vi "PositionerCapture_FocusedGaussLaw.vi"() -> ()   [LabVIEW 2011]
doc: "CONEX - CC Virtual Front Panel:\n\nThis is a sample of an application that can be built with the LabVIEW drivers.\n\nPress HOME / ENABLE in top left of panel to put stage in Ready state for motion."
uses:
  <vilib>/userDefined/High Color/IMAQdx.ctl
  <vilib>/Platform/TimedLoop/XDataNode/timing_clust.ctl
  <vilib>/Platform/TimedLoop/XDataNode/nitl_modes.ctl
  <vilib>/Platform/TimedLoop/XDataNode/wakeup.ctl
  <vilib>/Platform/TimedLoop/XDataNode/XDataNode.xnode
  <vilib>/Platform/TimedLoop/XDataNode/XDNodeRunTimeDep.lvlib
  <vilib>/vision/driver/NI_Vision_Acquisition_Software.lvlib
panel:
  out "Phase":bool
  out "Amp":bool
  in  "Next":bool
  out "Current noUnits":dbl caption="mm" format="%#_6f"
  in  "lambda":dbl caption="nm" format="%#_6f"
  in  "Units":string(combo)="mm"
  in  "Go0":bool
  in  "Zero position":dbl caption="mm" format="%#_6f"
  in  "Tare":bool
  out "Relative position":dbl caption="mm" format="%#_6f"
  in  "Folder's path where save the captures":path
  out "Image":T1(plugin-control)
  in  "(1) Go to:":dbl=1.0 caption="mm"
  out "Title":string
  in  "Set Max":bool
  in  "Set Min":bool
  in  "Max":dbl
  in  "Min":dbl
  in  "Set velocity":bool
  out "Stop cycle":bool=TRUE
  out "Title 2":string
  in  "Cycle":bool
  in  "Go2":bool
  in  "Go1":bool
  in  "(2) Go to:":dbl=1.0 caption="mm"
  in  "-":bool
  in  "+":bool
  in  "Step:":dbl caption="mm" format="%#_6f"
  out "Position History":dbl(graph)=1.5
  in  "Action":bool
  out "Stop polling":bool=TRUE
  out "Controller state description":string="STATUS"
  out "Velocity MAX":dbl=0.4
  out "Controller state":string="33"
  out "Positioner error":string="0000"
  in  "Velocity:":dbl format="%#_6f"
  in  "Exit":bool=TRUE
  out "Target position":dbl
  in  "Exit":bool
  in  "Position glissière":cluster{dbl, dbl}(slide) scale=0.0..25.0
  out "Current position":dbl caption="mm" format="%#_6f"
  # "mm/s"
  # "mm"
  # "Limits:"
  # "mm"
  # "(1)"
  # "(2)"
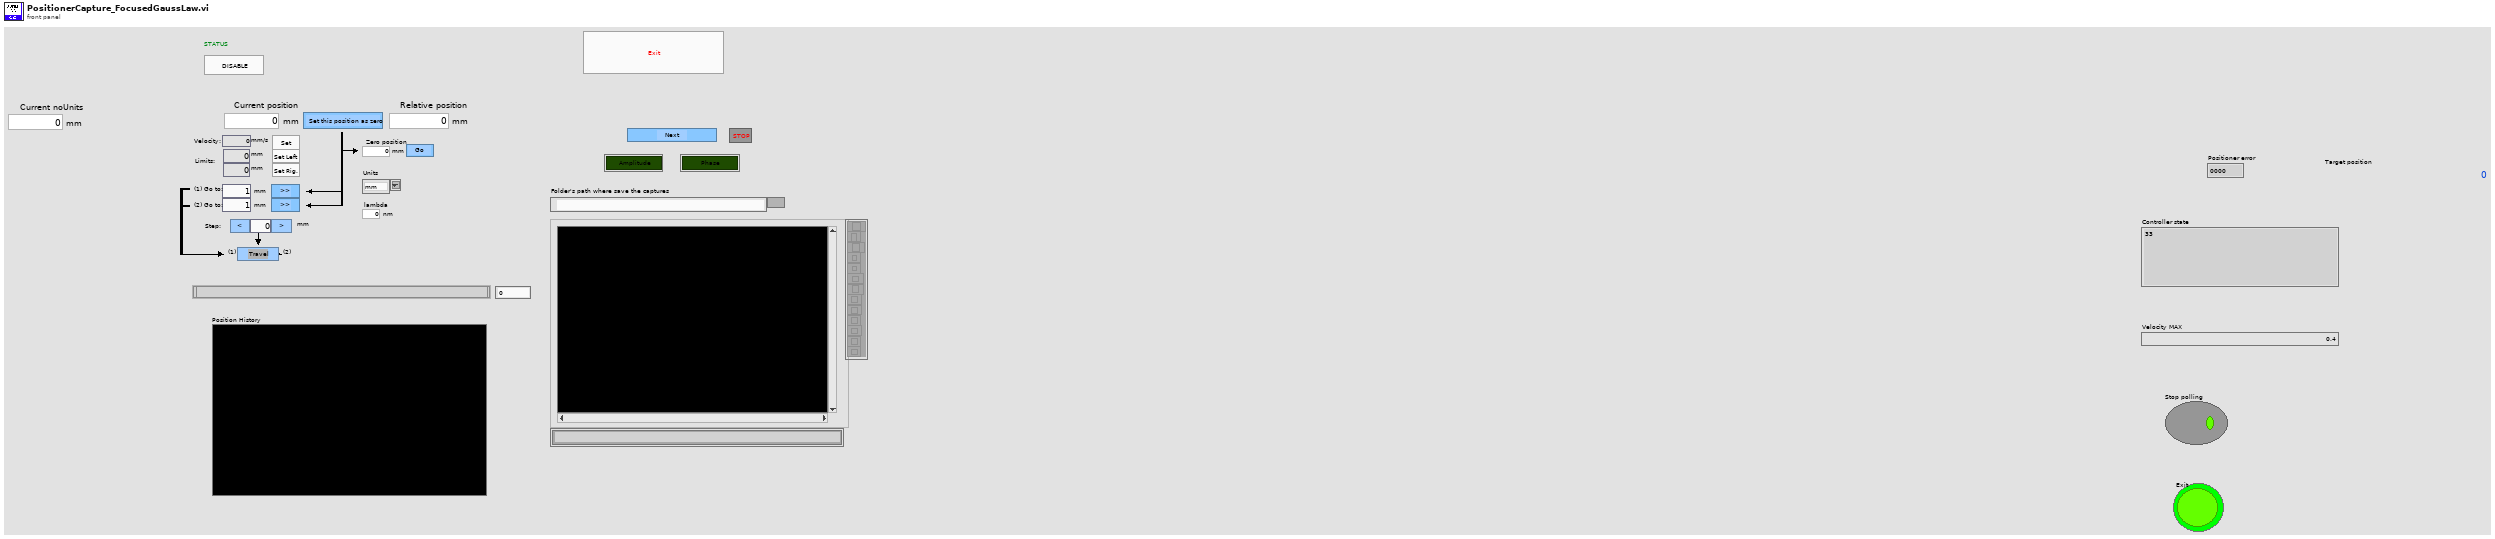
[diagram p1: front panel]
types:
  T1 = typedef "IMAQ Image.ctl" = refnum<image>
  T2 = typedef "IMAQdx.ctl" = refnum<k21>
  T3 = typedef "XDNodeRunTimeDep.lvlib/timing_clust.ctl" = cluster{"Expected End [f-1]":u64, "Actual End [f-1]":u64, "Finished Late? [f-1]":bool, "Expected End [i-1]":u64, "Actual End [i-1]":u64, "Finished Late? [i-1]":bool, "Expected Start [i]":u64, "Actual Start [i]":u64, "Expected Start [f]":u64, "Actual Start [f]":u64, "Source Name":string, "Structure Name":string, "Period":i64, "Deadline":i64, "Offset":i64, "Start":i64, "Priority":i32, "Timeout":i32, "Mode":T4, "Wakeup Reason":T5, "Error":errorcluster, "Source Type":string, "Secondary Source Type":string, "Global End Time":u64, "Global Start Time":u64, "Frame Duration":u64, "Iteration Duration":u64, "Assigned CPU":i32, "I/O Scan Engine Mode":u32}
  T4 = typedef "XDNodeRunTimeDep.lvlib/nitl_modes.ctl" = enum32{"No Change", "Process missed periods, maintain original phase", "Discard missed periods, maintain original phase", "Process missed periods, ignore original phase", "Discard missed periods, ignore original phase"}
  T5 = typedef "XDNodeRunTimeDep.lvlib/wakeup.ctl" = enum32{"Normal", "Aborted", "Asynchronous wakeup", "Timing source error", "Timed loop error", "Timeout"}
  T6 = cluster{"VISA resource name":refnum<visa-resource-name>, "Device name":string, "Controller address":i32, "error":errorcluster}
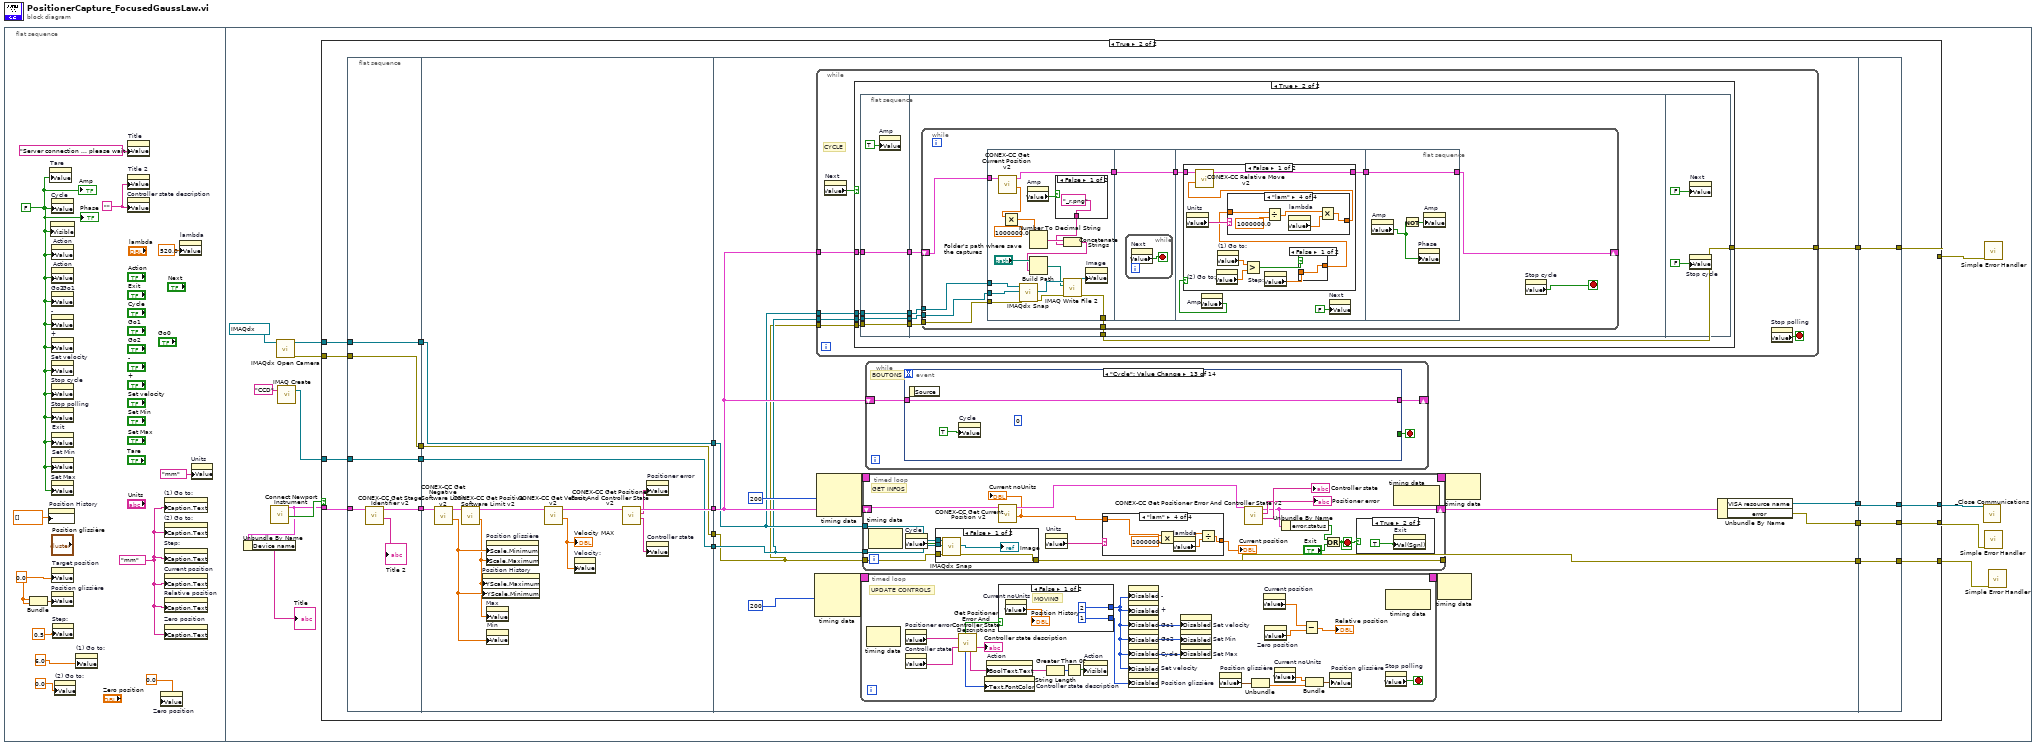
[diagram p0: block diagram]
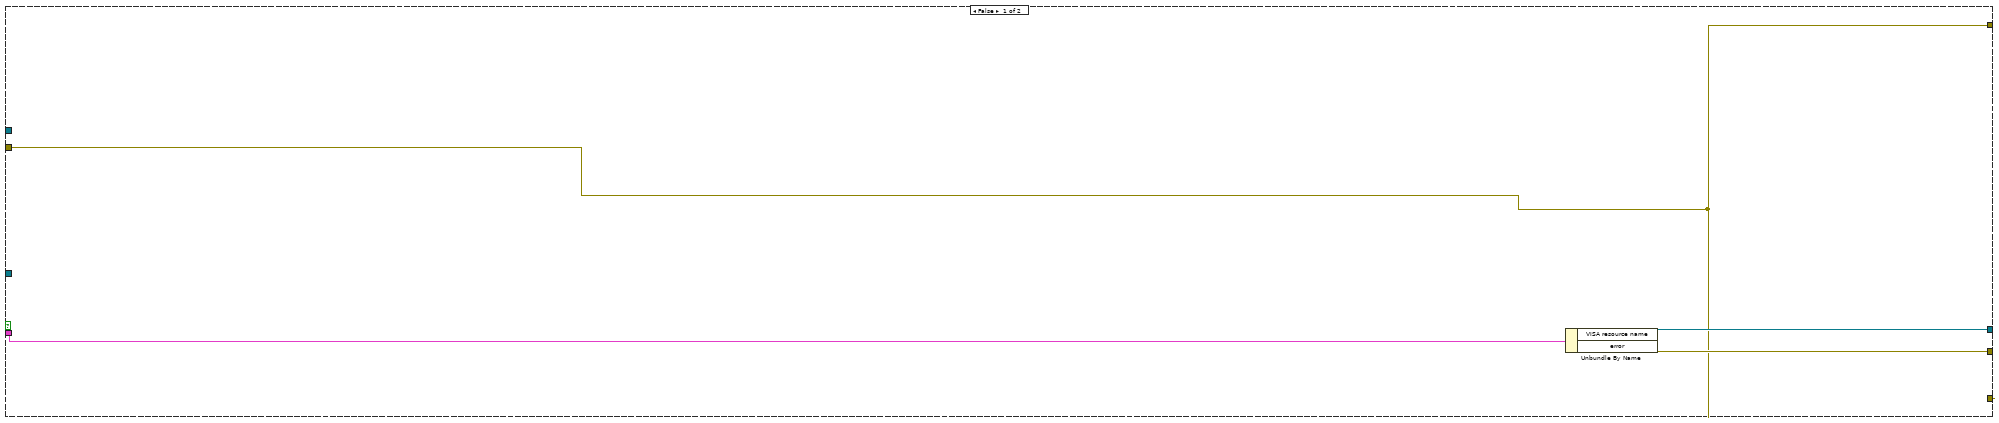
[diagram p2: hidden frame]
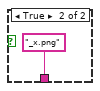
[diagram p4: hidden frame]
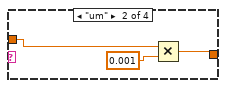
[diagram p6: hidden frame]
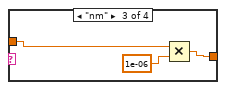
[diagram p7: hidden frame]
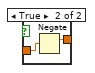
[diagram p8: hidden frame]
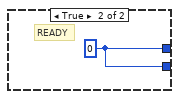
[diagram p10: hidden frame]
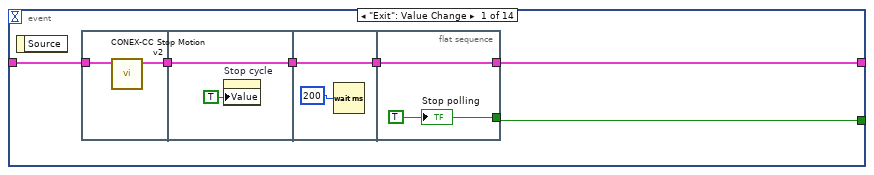
[diagram p11: hidden frame]
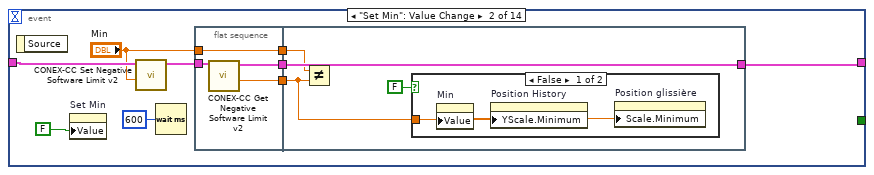
[diagram p12: hidden frame]
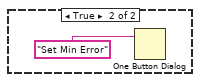
[diagram p13: hidden frame]
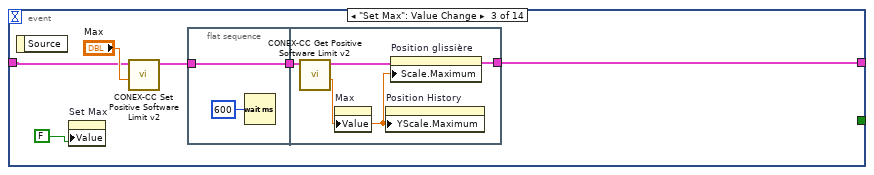
[diagram p14: hidden frame]
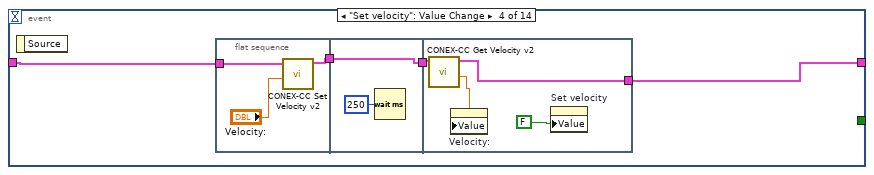
[diagram p15: hidden frame]
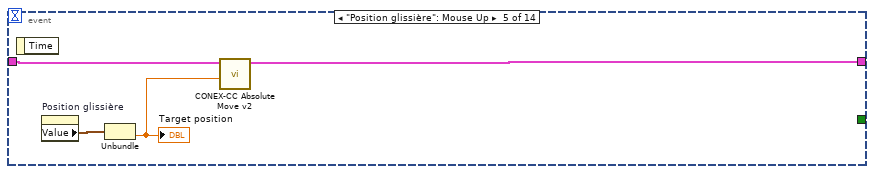
[diagram p16: hidden frame]
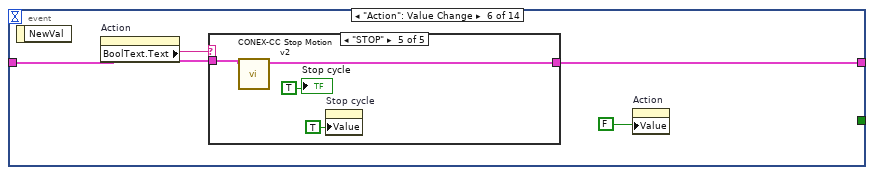
[diagram p17: hidden frame]
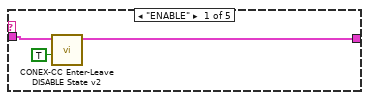
[diagram p18: hidden frame]
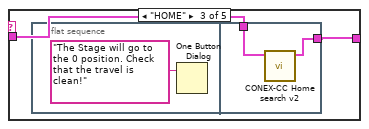
[diagram p20: hidden frame]
diagram:
  n1 = flat-sequence {
    frame #0 {
      w3 = "mm" ("Units")
      w1 = FALSE
      w12 = 0.0
      w11 = ""
      n2 = Bundle(w12, w12) -> (w13:cluster{dbl, dbl})  [unwired: 1 out]
      n3 = property on="Position History" class="WFChart (strict)"("History Data"=dbl[] [] ("Données d'historique")) -> ()  [unwired: 2 in, 2 out]
      n4 = property on="Tare" class="Bool (strict)"("Value"=w1) -> ()  [unwired: 2 in, 2 out]
      n5 = property on="Action" class="Bool (strict)"("Visible"=w1) -> ()  [unwired: 2 in, 2 out]
      n6 = property on="Cycle" class="Bool (strict)"("Value"=w1) -> ()  [unwired: 2 in, 2 out]
      n7 = property on="Action" class="Bool (strict)"("Value"=w1) -> ()  [unwired: 2 in, 2 out]
      n8 = property on="Go1" class="Bool (strict)"("Value"=w1) -> ()  [unwired: 2 in, 2 out]
      n9 = property on="Go2" class="Bool (strict)"("Value"=w1) -> ()  [unwired: 2 in, 2 out]
      n10 = property on="-" class="Bool (strict)"("Value"=w1) -> ()  [unwired: 2 in, 2 out]
      n11 = property on="+" class="Bool (strict)"("Value"=w1) -> ()  [unwired: 2 in, 2 out]
      n12 = property on="Set velocity" class="Bool (strict)"("Value"=w1) -> ()  [unwired: 2 in, 2 out]
      n13 = property on="Stop cycle" class="Bool (strict)"("Value"=w1) -> ()  [unwired: 2 in, 2 out]
      n14 = property on="Stop polling" class="Bool (strict)"("Value"=w1) -> ()  [unwired: 2 in, 2 out]
      n15 = property on="Exit" class="Bool (strict)"("Value"=w1) -> ()  [unwired: 2 in, 2 out]
      n16 = property on="Set Min" class="Bool (strict)"("Value"=w1) -> ()  [unwired: 2 in, 2 out]
      n17 = property on="Set Max" class="Bool (strict)"("Value"=w1) -> ()  [unwired: 2 in, 2 out]
      n18 = property on="Target position" class="DigNum (strict)"("Value"=w12) -> ()  [unwired: 2 in, 2 out]
      n19 = property on="Position glissière" class="Slide (strict)"("Value"=w13) -> ()  [unwired: 2 in, 2 out]
      n20 = property on="Step:" class="DigNum (strict)"("Value"=0.5 ("Step")) -> ()  [unwired: 2 in, 2 out]
      n21 = property on="(2) Go to:" class="DigNum (strict)"("Value"=0.0 ("Abs. Move 2")) -> ()  [unwired: 2 in, 2 out]
      n22 = property on="(1) Go to:" class="DigNum (strict)"("Value"=6.0 ("Abs. Move 1")) -> ()  [unwired: 2 in, 2 out]
      n23 = property on="Title" class="Str"("Value"="Server connection ... please wait." ("Title")) -> ()  [unwired: 2 in, 2 out]
      n24 = property on="Title 2" class="Str"("Value"=w11) -> ()  [unwired: 2 in, 2 out]
      n25 = property on="Controller state description" class="Str"("Value"=w11) -> ()  [unwired: 2 in, 2 out]
      n26 = property on="Zero position" class="DigNum (strict)"("Value"=0.0 ("Zero position")) -> ()  [unwired: 2 in, 2 out]
      n27 = property on="(1) Go to:" class="DigNum (strict)"("Caption.Text"=w3) -> ()  [unwired: 2 in, 2 out]
      n28 = property on="(2) Go to:" class="DigNum (strict)"("Caption.Text"=w3) -> ()  [unwired: 2 in, 2 out]
      n29 = property on="Step:" class="DigNum (strict)"("Caption.Text"=w3) -> ()  [unwired: 2 in, 2 out]
      n30 = property on="Current position" class="DigNum (strict)"("Caption.Text"=w3) -> ()  [unwired: 2 in, 2 out]
      n31 = property on="Relative position" class="DigNum (strict)"("Caption.Text"=w3) -> ()  [unwired: 2 in, 2 out]
      n32 = property on="Zero position" class="DigNum (strict)"("Caption.Text"=w3) -> ()  [unwired: 2 in, 2 out]
      n33 = property on="lambda" class="DigNum (strict)"("Value"=520.0 ("lambda")) -> ()  [unwired: 2 in, 2 out]
      n34 = property on="Units" class="CmbBox"("Value"="mm" ("Units")) -> ()  [unwired: 2 in, 2 out]
      "Amp" <- w1
      "Phase" <- w1
    }
    frame #1 {
      n35 = call <userlib>:"Connect Newport Instrument.vi"() -> ("Connected"=w23:bool, "Device Connection Cluster"=w22:T6)  [unwired: 7 in, 3 out]
      n36 = Unbundle By Name(w22) -> ("Device name"=→"Title":string)
      n37 = call <vilib>:"IMAQdx Open Camera.vi"("Session In"=T2 "Paraxial") -> ("error out"=w16:errorcluster, "Session Out"=w18:T2)  [unwired: 9 in]
      n38 = call "IMAQ Create"("Image Name"="CCD") -> ("New Image"=w17:T1)  [unwired: 4 in, 1 out]
      n39 = case shown="True" w23 {
        tunnel: [w28 w49] -> w25
        tunnel: w22 -> [w29 w47]
        tunnel: [w27 w43] -> w21
        tunnel: w18 -> [_ w41]
        tunnel: w17 -> [_ w38]
        tunnel: w16 -> [w26 w35]
        tunnel: [w26 w32] -> w15
        tunnel: [w26 w30] -> w14
        frame False {
          n40 = Unbundle By Name(w29) -> ("VISA resource name"=w27:refnum<visa-resource-name>, "error"=w28:errorcluster)
        }
        frame True {
          n41 = flat-sequence {
            tunnel: w47 -> [w55]
            tunnel: [w53] -> w46
            tunnel: [w52] -> w42
            tunnel: w41 -> [w52]
            tunnel: [w51] -> w39
            tunnel: w38 -> [w51]
            tunnel: [w50] -> w36
            tunnel: w35 -> [w50]
            tunnel: [w65] -> w48
            tunnel: w46 -> [w62]
            tunnel: w42 -> [w58]
            tunnel: [w58] -> w40
            tunnel: w39 -> [w57]
            tunnel: [w57] -> w37
            tunnel: w36 -> [w56]
            tunnel: [w56] -> w34
            tunnel: w48 -> [w74]
            tunnel: [w76] -> w45
            tunnel: [w75] -> w44
            tunnel: w40 -> [w73]
            tunnel: w37 -> [w72]
            tunnel: w34 -> [w71]
            tunnel: [w70] -> w33
            tunnel: [w69] -> w31
            tunnel: [w449] -> w49
            tunnel: w45 -> [w448]
            tunnel: w44 -> [w449]
            tunnel: [w448] -> w43
            tunnel: [w447] -> w32
            tunnel: w33 -> [w447]
            tunnel: [w446] -> w30
            tunnel: w31 -> [w446]
            frame #0 {
              n42 = call <userlib>:"CONEX-CC Get Stage Identifier v2.vi"("Connection Cluster in"=w55) -> ("Identifier"=→"Title 2":string, "Connection Cluster out"=w53:T6)  [unwired: 9 in]
            }
            frame #1 {
              n43 = call <userlib>:"CONEX-CC Get Negative Software Limit v2.vi"("Connection Cluster in"=w62) -> ("Left limit"=w67:dbl, "Connection Cluster out"=w61:T6)  [unwired: 9 in]
              n44 = call <userlib>:"CONEX-CC Get Positive Software Limit v2.vi"("Connection Cluster in"=w61) -> ("Right limit"=w66:dbl, "Connection Cluster out"=w60:T6)  [unwired: 9 in]
              n45 = property on="Position History" class="WFChart (strict)"("YScale.Maximum"=w66, "YScale.Minimum"=w67) -> ()  [unwired: 2 in, 2 out]
              n46 = property on="Position glissière" class="Slide (strict)"("Scale.Minimum"=w67, "Scale.Maximum"=w66) -> ()  [unwired: 2 in, 2 out]
              n47 = property on="Max" class="DigNum (strict)"("Value"=w66) -> ()  [unwired: 2 in, 2 out]
              n48 = property on="Min" class="DigNum (strict)"("Value"=w67) -> ()  [unwired: 2 in, 2 out]
              n49 = call <userlib>:"CONEX-CC Get Velocity v2.vi"("Connection Cluster in"=w60) -> ("Velocity"=w68:dbl, "Connection Cluster out"=w59:T6)  [unwired: 8 in, 1 out]
              "Velocity MAX" <- w68
              n50 = property on="Velocity:" class="DigNum (strict)"("Value"=w68) -> ()  [unwired: 2 in, 2 out]
              n51 = call <userlib>:"CONEX-CC Get Positioner Error And Controller State v2.vi"("Connection Cluster in"=w59) -> ("Controller state"=w63:string, "Positioner error"=w64:string, "Connection Cluster out"=w65:T6)  [unwired: 8 in]
              n52 = property on="Positioner error" class="Str"("Value"=w64) -> ()  [unwired: 2 in, 2 out]
              n53 = property on="Controller state" class="Str"("Value"=w63) -> ()  [unwired: 2 in, 2 out]
            }
            frame #2 {
              n54 = node-c288(i64 200 ("Période")) -> (w81:T3)  [unwired: 1 in, 1 out]
              n55 = while {
                tunnel: w74 -> [w90]
                tunnel: w73 -> [w87]
                tunnel: w72 -> [w86]
                tunnel: w71 -> [w85]
                tunnel: [w84] -> w69
                stop <- w89 stop-if-true
                # "CYCLE"
                n56 = property on="Next" class="Bool (strict)"() -> ("Value"=w88:bool)  [unwired: 2 in, 2 out]
                n57 = case shown="True" w88 {
                  tunnel: w90 -> [_ w97]
                  tunnel: w87 -> [_ w100]
                  tunnel: w86 -> [_ w99]
                  tunnel: w85 -> [w91 w98]
                  tunnel: [w91 w96] -> w84
                  frame False {
                  }
                  frame True {
                    n58 = flat-sequence {
                      tunnel: w97 -> [w102]
                      tunnel: w98 -> [w103]
                      tunnel: w99 -> [w104]
                      tunnel: w100 -> [w105]
                      tunnel: [w105] -> w95
                      tunnel: [w104] -> w94
                      tunnel: [w103] -> w93
                      tunnel: [w102] -> w92
                      tunnel: [w106] -> w96
                      tunnel: w95 -> [w110]
                      tunnel: w94 -> [w109]
                      tunnel: w93 -> [w108]
                      tunnel: w92 -> [w107]
                      frame #0 {
                        n59 = property on="Amp" class="Bool (strict)"("Value"=TRUE ("Amp")) -> ()  [unwired: 2 in, 2 out]
                      }
                      frame #1 {
                        n60 = while {
                          shift-right: [w112] -> _
                          shift-left: w107 -> [w120]
                          tunnel: w110 -> [w119]
                          tunnel: w109 -> [w115]
                          tunnel: w108 -> [w118]
                          tunnel: [w113] -> w106
                          stop <- w111 stop-if-true
                          n61 = flat-sequence {
                            tunnel: w120 -> [w132]
                            tunnel: w119 -> [w130]
                            tunnel: w115 -> [w129]
                            tunnel: w118 -> [w128]
                            tunnel: [w131] -> w116
                            tunnel: [w121] -> w113
                            tunnel: [w141] -> w117
                            tunnel: w116 -> [w141]
                            tunnel: w117 -> [w146]
                            tunnel: [w145] -> w114
                            tunnel: [w174] -> w112
                            tunnel: w114 -> [w174]
                            frame #0 {
                              n62 = call <userlib>:"CONEX-CC Get Current Position v2.vi"("Connection Cluster in"=w132) -> ("Current position"=w124:dbl, "Connection Cluster out"=w131:T6)  [unwired: 8 in, 1 out]
                              n63 = Multiply(x=w124, y=1000000.0) -> (x*y=w137:dbl)
                              n64 = call <vilib>:"IMAQdx Snap.vi"("error in"=w128, "Image In"=w129, "Session In"=w130) -> ("error out"=w127:errorcluster, "Image Out"=w133:T1)  [unwired: 6 in, 1 out]
                              n65 = property on="Amp" class="Bool (strict)"() -> ("Value"=w123:bool)  [unwired: 2 in, 2 out]
                              n66 = Number To Decimal String(number=w137) -> (decimal integer string=w138:string)  [unwired: 1 in]
                              n67 = case shown="False" w123 {
                                tunnel: ["_r.png" ("string") "_x.png" ("string")] -> w122
                                frame False {
                                }
                                frame True {
                                }
                              }
                              n68 = Concatenate Strings(w138, w122) -> (w125:string)
                              n69 = Build Path(base path="Folder's path where save the captures", name or relative path=w125) -> (appended path=w126:path)
                              n70 = call-poly "IMAQ Write File 2"("error in (no error)"=w127, "File Path"=w126, "Image"=w133) -> ("error out"=w121:errorcluster, "Image Out (duplicate)"=w134:T1)  [unwired: 7 in]
                              n71 = property on="Image" class="ImageControl"("Value"=w134) -> ()  [unwired: 2 in, 2 out]
                            }
                            frame #1 {
                              n72 = while {
                                stop <- w142 stop-if-true
                                n73 = property on="Next" class="Bool (strict)"() -> ("Value"=w142:bool)  [unwired: 2 in, 2 out]
                              }
                            }
                            frame #2 {
                              n74 = property on="Amp" class="Bool (strict)"() -> ("Value"=w143:bool)  [unwired: 2 in, 2 out]
                              n75 = case shown="False" w143 {
                                tunnel: w146 -> [w149 w171]
                                tunnel: [w148 w171] -> w145
                                frame False {
                                n76 = property on="Units" class="CmbBox"() -> ("Value"=w155:string)  [unwired: 2 in, 2 out]
                                n77 = property on="(2) Go to:" class="DigNum (strict)"() -> ("Value"=w150:dbl)  [unwired: 2 in, 2 out]
                                n78 = property on="(1) Go to:" class="DigNum (strict)"() -> ("Value"=w151:dbl)  [unwired: 2 in, 2 out]
                                n79 = Greater?(x=w151, y=w150) -> (0:w152:bool)
                                n80 = property on="Step:" class="DigNum (strict)"() -> ("Value"=w153:dbl)  [unwired: 2 in, 2 out]
                                n81 = case shown="False" w152 {
                                tunnel: [w168 w169] -> w154
                                tunnel: w153 -> [w168 w170]
                                frame False {
                                }
                                frame True {
                                n82 = Negate(x=w170) -> (-x=w169:dbl)
                                }
                                }
                                n83 = case shown="\"lam\"" w155 {
                                tunnel: [w156 w158 w161 w164] -> w147
                                tunnel: w154 -> [w156 w157 w160 w163]
                                frame "mm", Default {
                                }
                                frame "um" {
                                n84 = Multiply(x=w157, y=0.001) -> (x*y=w158:dbl)
                                }
                                frame "nm" {
                                n85 = Multiply(x=w160, y=1e-06) -> (x*y=w161:dbl)
                                }
                                frame "lam" {
                                n86 = Divide(x=w163, y=1000000.0) -> (x/y=w166:dbl)
                                n87 = property on="lambda" class="DigNum (strict)"() -> ("Value"=w165:dbl)  [unwired: 2 in, 2 out]
                                n88 = Multiply(x=w166, y=w165) -> (x*y=w164:dbl)
                                }
                                }
                                n89 = call <userlib>:"CONEX-CC Relative Move v2.vi"("Relative displacement"=w147, "Connection Cluster in"=w149) -> ("Connection Cluster out"=w148:T6)  [unwired: 9 in]
                                }
                                frame True {
                                }
                              }
                              n90 = property on="Next" class="Bool (strict)"("Value"=FALSE ("Next")) -> ()  [unwired: 2 in, 2 out]
                            }
                            frame #3 {
                              n91 = property on="Amp" class="Bool (strict)"() -> ("Value"=w173:bool)  [unwired: 2 in, 2 out]
                              n92 = Not(x=w173) -> (.not. x?=w172:bool)
                              n93 = property on="Phase" class="Bool (strict)"("Value"=w173) -> ()  [unwired: 2 in, 2 out]
                              n94 = property on="Amp" class="Bool (strict)"("Value"=w172) -> ()  [unwired: 2 in, 2 out]
                            }
                          }
                          n95 = property on="Stop cycle" class="Bool (strict)"() -> ("Value"=w111:bool)  [unwired: 2 in, 2 out]
                        }
                      }
                      frame #2 {
                        n96 = property on="Next" class="Bool (strict)"("Value"=FALSE ("Cycle")) -> ()  [unwired: 2 in, 2 out]
                        n97 = property on="Stop cycle" class="Bool (strict)"("Value"=FALSE ("Cycle")) -> ()  [unwired: 2 in, 2 out]
                      }
                    }
                  }
                }
                n98 = property on="Stop polling" class="Bool (strict)"() -> ("Value"=w89:bool)  [unwired: 2 in, 2 out]
              }
              n99 = node-c288(i64 200 ("Période")) -> (w83:T3)  [unwired: 1 in, 1 out]
              n100 = timed-loop {
                timing: w81 -> [_]
                timing-out: [_] -> w80
                stop <- w185 stop-if-true
                # "UPDATE CONTROLS"
                n101 = node-c288() -> ()  [unwired: 2 out]
                n102 = property on="Positioner error" class="Str"() -> ("Value"=w194:string)  [unwired: 2 in, 2 out]
                n103 = property on="Controller state" class="Str"() -> ("Value"=w193:string)  [unwired: 2 in, 2 out]
                n104 = call <userlib>:"Get Positioner Error And Controller State Descriptions.vi"("Controller state"=w193, "Positioner error"=w194) -> ("Color"=w191:u32, "Action name"=w190:string, "Controller state description"=→"Controller state description":string, "IsReady?"=w187:bool)  [unwired: 2 out]
                n105 = property on="Controller state description" class="Str"("Text.FontColor"=w191) -> ()  [unwired: 2 in, 2 out]
                n106 = property on="Action" class="Bool (strict)"("BoolText.Text"=w190) -> ()  [unwired: 2 in, 2 out]
                n107 = case shown="False" w187 {
                  tunnel: [u8 2 w198] -> w184
                  tunnel: [u8 1 w198] -> w186
                  frame False {
                    # "MOVING"
                    n108 = property on="Current noUnits" class="DigNum (strict)"() -> ("Value"=→"Position History":dbl)  [unwired: 2 in, 2 out]
                  }
                  frame True {
                    w198 = u8 0
                    # "READY"
                  }
                }
                n109 = String Length(string=w190) -> (length=w189:i32)
                n110 = Greater Than 0?(x=w189) -> (x > 0?=w188:bool)
                n111 = property on="Action" class="Bool (strict)"("Visible"=w188) -> ()  [unwired: 2 in, 2 out]
                n112 = property on="-" class="Bool (strict)"("Disabled"=w184) -> ()  [unwired: 2 in, 2 out]
                n113 = property on="+" class="Bool (strict)"("Disabled"=w184) -> ()  [unwired: 2 in, 2 out]
                n114 = property on="Go1" class="Bool (strict)"("Disabled"=w184) -> ()  [unwired: 2 in, 2 out]
                n115 = property on="Go2" class="Bool (strict)"("Disabled"=w184) -> ()  [unwired: 2 in, 2 out]
                n116 = property on="Cycle" class="Bool (strict)"("Disabled"=w184) -> ()  [unwired: 2 in, 2 out]
                n117 = property on="Set velocity" class="Bool (strict)"("Disabled"=w184) -> ()  [unwired: 2 in, 2 out]
                n118 = property on="Position glissière" class="Slide (strict)"("Disabled"=w186) -> ()  [unwired: 2 in, 2 out]
                n119 = property on="Set velocity" class="Bool (strict)"("Disabled"=w184) -> ()  [unwired: 2 in, 2 out]
                n120 = property on="Set Min" class="Bool (strict)"("Disabled"=w184) -> ()  [unwired: 2 in, 2 out]
                n121 = property on="Set Max" class="Bool (strict)"("Disabled"=w184) -> ()  [unwired: 2 in, 2 out]
                n122 = property on="Position glissière" class="Slide (strict)"() -> ("Value"=w182:cluster{dbl, dbl})  [unwired: 2 in, 2 out]
                n123 = Unbundle(w182) -> (w181:dbl)  [unwired: 1 out]
                n124 = property on="Current position" class="DigNum (strict)"() -> ("Value"=w177:dbl)  [unwired: 2 in, 2 out]
                n125 = property on="Zero position" class="DigNum (strict)"() -> ("Value"=w178:dbl)  [unwired: 2 in, 2 out]
                n126 = property on="Current noUnits" class="DigNum (strict)"() -> ("Value"=w179:dbl)  [unwired: 2 in, 2 out]
                n127 = Subtract(x=w177, y=w178) -> (x-y=→"Relative position":dbl)
                n128 = Bundle("Value"=w179, w181) -> (w183:cluster{"Value":dbl, dbl})  [unwired: 1 out]
                n129 = property on="Position glissière" class="Slide (strict)"("Value"=w183) -> ()  [unwired: 2 in, 2 out]
                n130 = node-c288() -> ()  [unwired: 2 out]
                n131 = property on="Stop polling" class="Bool (strict)"() -> ("Value"=w185:bool)  [unwired: 2 in, 2 out]
              }
              n132 = timed-loop {
                timing: w83 -> [_]
                timing-out: [_] -> w82
                shift-right: [w410] -> w77
                shift-left: w74 -> [w420]
                tunnel: w73 -> [w419]
                tunnel: w72 -> [w418]
                tunnel: w71 -> [w417]
                tunnel: [w416] -> w70
                stop <- w413 stop-if-true
                # "GET INFOS"
                n133 = node-c288() -> ()  [unwired: 2 out]
                n134 = property on="Cycle" class="Bool (strict)"() -> ("Value"=w415:bool)  [unwired: 2 in, 2 out]
                n135 = case shown="False" w415 {
                  tunnel: w419 -> [w437 _]
                  tunnel: w418 -> [w436 _]
                  tunnel: w417 -> [w435 w438]
                  tunnel: [w433 w438] -> w416
                  frame False {
                    n136 = call <vilib>:"IMAQdx Snap.vi"("error in"=w435, "Image In"=w436, "Session In"=w437) -> ("error out"=w433:errorcluster, "Image Out"=→"Image":T1)  [unwired: 6 in, 1 out]
                  }
                  frame True {
                  }
                }
                n137 = call <userlib>:"CONEX-CC Get Current Position v2.vi"("Connection Cluster in"=w420) -> ("Current position"=w406:dbl, "Connection Cluster out"=w407:T6)  [unwired: 8 in, 1 out]
                "Current noUnits" <- w406
                n138 = property on="Units" class="CmbBox"() -> ("Value"=w405:string)  [unwired: 2 in, 2 out]
                n139 = case shown="\"lam\"" w405 {
                  tunnel: [w421 w422 w425 w428] -> w409
                  tunnel: w406 -> [w421 w423 w426 w429]
                  frame "mm", Default {
                  }
                  frame "um" {
                    n140 = Multiply(x=w423, y=1000.0) -> (x*y=w422:dbl)
                  }
                  frame "nm" {
                    n141 = Multiply(x=w426, y=1000000.0) -> (x*y=w425:dbl)
                  }
                  frame "lam" {
                    n142 = Multiply(x=w429, y=1000000.0) -> (x*y=w432:dbl)
                    n143 = property on="lambda" class="DigNum (strict)"() -> ("Value"=w430:dbl)  [unwired: 2 in, 2 out]
                    n144 = Divide(x=w432, y=w430) -> (x/y=w428:dbl)
                  }
                }
                "Current position" <- w409
                n145 = call <userlib>:"CONEX-CC Get Positioner Error And Controller State v2.vi"("Connection Cluster in"=w407) -> ("Controller state"=→"Controller state":string, "Positioner error"=→"Positioner error":string, "Connection Cluster out"=w410:T6)  [unwired: 8 in]
                n146 = Unbundle By Name(w410) -> ("error.status"=w408:bool)
                n147 = Or(x=w408, y="Exit") -> (x .or. y?=w413:bool)
                n148 = case shown="True" w413 {
                  frame False {
                  }
                  frame True {
                    n149 = property on="Exit" class="Bool (strict)"("Val(Sgnl)"=TRUE) -> ()  [unwired: 2 in, 2 out]
                  }
                }
                n150 = node-c288() -> ()  [unwired: 2 out]
              }
              n151 = while {
                shift-right: [w207] -> _
                shift-left: w74 -> [w206]
                stop <- w205 stop-if-true
                # "BOUTONS"
                n152 = event shown="[12] \"Cycle\": Value Change" {
                  selector: _ -> [_ _ _ _ _ _ _ _ _ _ _ _ _ _]
                  dyn-events: _ -> [_ _ _ _ _ _ _ _ _ _ _ _ _ _]
                  timeout: _ -> [_ _ _ _ _ _ _ _ _ _ _ _ _ _]
                  tunnel: [w211 _ _ _ _ _ _ _ _ _ _ _ _ _] -> w205
                  tunnel: w206 -> [w208 w228 w242 w255 w267 w271 w290 w311 w332 w352 w369 w385 w387 w396]
                  tunnel: [w213 w227 w241 w252 w266 w270 w289 w312 w331 w351 w370 w385 w387 w396] -> w207
                  event "Exit": Value Change {
                    n153 = event-data() -> ()  [unwired: 2 out]
                    n154 = flat-sequence {
                      tunnel: [w215] -> w212
                      tunnel: w208 -> [w214]
                      tunnel: w212 -> [w217]
                      tunnel: [w217] -> w210
                      tunnel: w210 -> [w219]
                      tunnel: [w219] -> w209
                      tunnel: [w221] -> w213
                      tunnel: w209 -> [w221]
                      tunnel: [w220] -> w211
                      frame #0 {
                        n155 = call <userlib>:"CONEX-CC Stop Motion v2.vi"("Connection Cluster in"=w214) -> ("Connection Cluster out"=w215:T6)  [unwired: 10 in]
                      }
                      frame #1 {
                        n156 = property on="Stop cycle" class="Bool (strict)"("Value"=TRUE) -> ()  [unwired: 2 in, 2 out]
                      }
                      frame #2 {
                        n157 = Wait (ms)(milliseconds to wait=u32 200 ("attente (ms)")) -> ()  [unwired: 1 out]
                      }
                      frame #3 {
                        w220 = TRUE
                        "Stop polling" <- w220
                      }
                    }
                  }
                  event "Set Min": Value Change {
                    n158 = event-data() -> ()  [unwired: 2 out]
                    n159 = property on="Set Min" class="Bool (strict)"("Value"=FALSE ("Set Min")) -> ()  [unwired: 2 in, 2 out]
                    n160 = call <userlib>:"CONEX-CC Set Negative Software Limit v2.vi"("Negative limit (left)"="Min", "Connection Cluster in"=w228) -> ("Connection Cluster out"=w230:T6)  [unwired: 9 in]
                    n161 = Wait (ms)(milliseconds to wait=u32 600 ("attente (ms)")) -> ()  [unwired: 1 out]
                    n162 = flat-sequence {
                      tunnel: w230 -> [w234]
                      tunnel: [w233] -> w225
                      tunnel: [w232] -> w224
                      tunnel: "Min" -> [w232]
                      tunnel: [w231] -> w222
                      tunnel: [w238] -> w227
                      tunnel: w225 -> [w238]
                      tunnel: w224 -> [w237]
                      tunnel: w222 -> [w235]
                      frame #0 {
                        n163 = call <userlib>:"CONEX-CC Get Negative Software Limit v2.vi"("Connection Cluster in"=w234) -> ("Left limit"=w231:dbl, "Connection Cluster out"=w233:T6)  [unwired: 9 in]
                      }
                      frame #1 {
                        n164 = Not Equal?(x=w237, y=w235) -> ()  [unwired: 1 out]
                        n165 = case shown="False" FALSE {
                          tunnel: w235 -> [w239 _]
                          frame False {
                            n166 = property on="Min" class="DigNum (strict)"("Value"=w239) -> ()  [unwired: 2 in, 2 out]
                            n167 = property on="Position History" class="WFChart (strict)"("YScale.Minimum"=w239) -> ()  [unwired: 2 in, 2 out]
                            n168 = property on="Position glissière" class="Slide (strict)"("Scale.Minimum"=w239) -> ()  [unwired: 2 in, 2 out]
                          }
                          frame True {
                            n169 = One Button Dialog(message="Set Min Error") -> ()  [unwired: 1 in, 1 out]
                          }
                        }
                      }
                    }
                  }
                  event "Set Max": Value Change {
                    n170 = event-data() -> ()  [unwired: 2 out]
                    n171 = property on="Set Max" class="Bool (strict)"("Value"=FALSE ("Set Max")) -> ()  [unwired: 2 in, 2 out]
                    n172 = call <userlib>:"CONEX-CC Set Positive Software Limit v2.vi"("Positive limit (right)"="Max", "Connection Cluster in"=w242) -> ("Connection Cluster out"=w246:T6)  [unwired: 9 in]
                    n173 = flat-sequence {
                      tunnel: w246 -> [w248]
                      tunnel: [w248] -> w243
                      tunnel: [w251] -> w241
                      tunnel: w243 -> [w249]
                      frame #0 {
                        n174 = Wait (ms)(milliseconds to wait=u32 600 ("attente (ms)")) -> ()  [unwired: 1 out]
                      }
                      frame #1 {
                        n175 = call <userlib>:"CONEX-CC Get Positive Software Limit v2.vi"("Connection Cluster in"=w249) -> ("Right limit"=w250:dbl, "Connection Cluster out"=w251:T6)  [unwired: 9 in]
                        n176 = property on="Max" class="DigNum (strict)"("Value"=w250) -> ()  [unwired: 2 in, 2 out]
                        n177 = property on="Position History" class="WFChart (strict)"("YScale.Maximum"=w250) -> ()  [unwired: 2 in, 2 out]
                        n178 = property on="Position glissière" class="Slide (strict)"("Scale.Maximum"=w250) -> ()  [unwired: 2 in, 2 out]
                      }
                    }
                  }
                  event "Set velocity": Value Change {
                    n179 = event-data() -> ()  [unwired: 2 out]
                    n180 = flat-sequence {
                      tunnel: w255 -> [w257]
                      tunnel: [w256] -> w253
                      tunnel: [w260] -> w254
                      tunnel: w253 -> [w260]
                      tunnel: w254 -> [w264]
                      tunnel: [w263] -> w252
                      frame #0 {
                        n181 = call <userlib>:"CONEX-CC Set Velocity v2.vi"("Velocity"="Velocity:", "Connection Cluster in"=w257) -> ("Connection Cluster out"=w256:T6)  [unwired: 9 in]
                      }
                      frame #1 {
                        n182 = Wait (ms)(milliseconds to wait=u32 250 ("attente (ms)")) -> ()  [unwired: 1 out]
                      }
                      frame #2 {
                        n183 = call <userlib>:"CONEX-CC Get Velocity v2.vi"("Connection Cluster in"=w264) -> ("Velocity"=w262:dbl, "Connection Cluster out"=w263:T6)  [unwired: 8 in, 1 out]
                        n184 = property on="Velocity:" class="DigNum (strict)"("Value"=w262) -> ()  [unwired: 2 in, 2 out]
                        n185 = property on="Set velocity" class="Bool (strict)"("Value"=FALSE ("Set velocity")) -> ()  [unwired: 2 in, 2 out]
                      }
                    }
                  }
                  event "Position glissière": Mouse Up {
                    n186 = event-data() -> ()  [unwired: 2 out]
                    n187 = property on="Position glissière" class="Slide (strict)"() -> ("Value"=w268:cluster{dbl, dbl})  [unwired: 2 in, 2 out]
                    n188 = Unbundle(w268) -> (w265:dbl)  [unwired: 1 out]
                    "Target position" <- w265
                    n189 = call <userlib>:"CONEX-CC Absolute Move v2.vi"("Target position"=w265, "Connection Cluster in"=w267) -> ("Connection Cluster out"=w266:T6)  [unwired: 5 in, 2 out]
                  }
                  event "Action": Value Change {
                    n190 = event-data() -> ()  [unwired: 2 out]
                    n191 = property on="Action" class="Bool (strict)"() -> ("BoolText.Text"=w272:string)  [unwired: 2 in, 2 out]
                    n192 = case shown="\"STOP\"" w272 {
                      tunnel: w271 -> [w274 w276 w278 w284 w286]
                      tunnel: [w273 w276 w277 w283 w288] -> w270
                      frame "ENABLE" {
                        n193 = call <userlib>:"CONEX-CC Enter-Leave DISABLE State v2.vi"("Ready? (false=DISABLE true=READY)"=TRUE ("Flag (false=DISABLE true=READY)"), "Connection Cluster in"=w274) -> ("Connection Cluster out"=w273:T6)  [unwired: 7 in]
                      }
                      frame Default {
                      }
                      frame "HOME" {
                        n194 = flat-sequence {
                          tunnel: w278 -> [w281]
                          tunnel: [w280] -> w277
                          frame #0 {
                            n195 = One Button Dialog(message="The Stage will go to the 0 position. Check that the travel is clean!") -> ()  [unwired: 1 in, 1 out]
                          }
                          frame #1 {
                            n196 = call <userlib>:"CONEX-CC Home search v2.vi"("Connection Cluster in"=w281) -> ("Connection Cluster out"=w280:T6)  [unwired: 5 in, 3 out]
                          }
                        }
                      }
                      frame "DISABLE" {
                        n197 = call <userlib>:"CONEX-CC Enter-Leave DISABLE State v2.vi"("Ready? (false=DISABLE true=READY)"=FALSE ("Flag (false=DISABLE true=READY)"), "Connection Cluster in"=w284) -> ("Connection Cluster out"=w283:T6)  [unwired: 7 in]
                      }
                      frame "STOP" {
                        n198 = call <userlib>:"CONEX-CC Stop Motion v2.vi"("Connection Cluster in"=w286) -> ("Connection Cluster out"=w288:T6)  [unwired: 10 in]
                        n199 = property on="Stop cycle" class="Bool (strict)"("Value"=TRUE) -> ()  [unwired: 2 in, 2 out]
                        "Stop cycle" <- TRUE ("Stop cycle")
                      }
                    }
                    n200 = property on="Action" class="Bool (strict)"("Value"=FALSE) -> ()  [unwired: 2 in, 2 out]
                  }
                  event "-": Value Change {
                    n201 = event-data() -> ()  [unwired: 2 out]
                    n202 = property on="-" class="Bool (strict)"("Value"=FALSE ("-")) -> ()  [unwired: 2 in, 2 out]
                    n203 = Negate(x="Step:") -> (-x=w293:dbl)
                    n204 = property on="Units" class="CmbBox"() -> ("Value"=w291:string)  [unwired: 2 in, 2 out]
                    n205 = case shown="\"lam\"" w291 {
                      tunnel: [w296 w297 w300 w303] -> w292
                      tunnel: w293 -> [w296 w298 w301 w307]
                      frame "mm", Default {
                      }
                      frame "um" {
                        n206 = Multiply(x=w298, y=0.001) -> (x*y=w297:dbl)
                      }
                      frame "nm" {
                        n207 = Multiply(x=w301, y=1e-06) -> (x*y=w300:dbl)
                      }
                      frame "lam" {
                        n208 = Divide(x=w307, y=1000000.0) -> (x/y=w305:dbl)
                        n209 = property on="lambda" class="DigNum (strict)"() -> ("Value"=w304:dbl)  [unwired: 2 in, 2 out]
                        n210 = Multiply(x=w305, y=w304) -> (x*y=w303:dbl)
                      }
                    }
                    n211 = call <userlib>:"CONEX-CC Relative Move v2.vi"("Relative displacement"=w292, "Connection Cluster in"=w290) -> ("Connection Cluster out"=w289:T6)  [unwired: 9 in]
                  }
                  event "+": Value Change {
                    n212 = event-data() -> ()  [unwired: 2 out]
                    n213 = property on="+" class="Bool (strict)"("Value"=FALSE ("+")) -> ()  [unwired: 2 in, 2 out]
                    n214 = property on="Step:" class="DigNum (strict)"() -> ("Value"=w310:dbl)  [unwired: 2 in, 2 out]
                    n215 = property on="Units" class="CmbBox"() -> ("Value"=w309:string)  [unwired: 2 in, 2 out]
                    n216 = case shown="\"lam\"" w309 {
                      tunnel: [w314 w315 w318 w321] -> w308
                      tunnel: w310 -> [w314 w316 w319 w325]
                      frame "mm", Default {
                      }
                      frame "um" {
                        n217 = Multiply(x=w316, y=0.001) -> (x*y=w315:dbl)
                      }
                      frame "nm" {
                        n218 = Multiply(x=w319, y=1e-06) -> (x*y=w318:dbl)
                      }
                      frame "lam" {
                        n219 = Divide(x=w325, y=1000000.0) -> (x/y=w323:dbl)
                        n220 = property on="lambda" class="DigNum (strict)"() -> ("Value"=w322:dbl)  [unwired: 2 in, 2 out]
                        n221 = Multiply(x=w323, y=w322) -> (x*y=w321:dbl)
                      }
                    }
                    n222 = call <userlib>:"CONEX-CC Relative Move v2.vi"("Relative displacement"=w308, "Connection Cluster in"=w311) -> ("Connection Cluster out"=w312:T6)  [unwired: 9 in]
                  }
                  event "Go1": Value Change {
                    n223 = event-data() -> ()  [unwired: 2 out]
                    n224 = property on="Go1" class="Bool (strict)"("Value"=FALSE ("Go1")) -> ()  [unwired: 2 in, 2 out]
                    n225 = property on="Zero position" class="DigNum (strict)"() -> ("Value"=w329:dbl)  [unwired: 2 in, 2 out]
                    n226 = property on="Units" class="CmbBox"() -> ("Value"=w330:string)  [unwired: 2 in, 2 out]
                    n227 = Add(x="(1) Go to:", y=w329) -> (x+y=w327:dbl)
                    n228 = case shown="\"lam\"" w330 {
                      tunnel: [w334 w335 w338 w341] -> w326
                      tunnel: w327 -> [w334 w336 w339 w345]
                      frame "mm", Default {
                      }
                      frame "um" {
                        n229 = Multiply(x=w336, y=0.001) -> (x*y=w335:dbl)
                      }
                      frame "nm" {
                        n230 = Multiply(x=w339, y=1e-06) -> (x*y=w338:dbl)
                      }
                      frame "lam" {
                        n231 = Divide(x=w345, y=1000000.0) -> (x/y=w343:dbl)
                        n232 = property on="lambda" class="DigNum (strict)"() -> ("Value"=w342:dbl)  [unwired: 2 in, 2 out]
                        n233 = Multiply(x=w343, y=w342) -> (x*y=w341:dbl)
                      }
                    }
                    n234 = call <userlib>:"CONEX-CC Absolute Move v2.vi"("Target position"=w326, "Connection Cluster in"=w332) -> ("Connection Cluster out"=w331:T6)  [unwired: 5 in, 2 out]
                  }
                  event "Go2": Value Change {
                    n235 = event-data() -> ()  [unwired: 2 out]
                    n236 = property on="Go2" class="Bool (strict)"("Value"=FALSE ("Go2")) -> ()  [unwired: 2 in, 2 out]
                    n237 = property on="Zero position" class="DigNum (strict)"() -> ("Value"=w349:dbl)  [unwired: 2 in, 2 out]
                    n238 = property on="Units" class="CmbBox"() -> ("Value"=w350:string)  [unwired: 2 in, 2 out]
                    n239 = Add(x="(2) Go to:", y=w349) -> (x+y=w347:dbl)
                    n240 = case shown="\"lam\"" w350 {
                      tunnel: [w354 w356 w359 w362] -> w346
                      tunnel: w347 -> [w354 w355 w358 w361]
                      frame "mm", Default {
                      }
                      frame "um" {
                        n241 = Multiply(x=w355, y=0.001) -> (x*y=w356:dbl)
                      }
                      frame "nm" {
                        n242 = Multiply(x=w358, y=1e-06) -> (x*y=w359:dbl)
                      }
                      frame "lam" {
                        n243 = Divide(x=w361, y=1000000.0) -> (x/y=w364:dbl)
                        n244 = property on="lambda" class="DigNum (strict)"() -> ("Value"=w363:dbl)  [unwired: 2 in, 2 out]
                        n245 = Multiply(x=w364, y=w363) -> (x*y=w362:dbl)
                      }
                    }
                    n246 = call <userlib>:"CONEX-CC Absolute Move v2.vi"("Target position"=w346, "Connection Cluster in"=w352) -> ("Connection Cluster out"=w351:T6)  [unwired: 5 in, 2 out]
                  }
                  event "Go0": Value Change {
                    n247 = event-data() -> ()  [unwired: 2 out]
                    n248 = property on="Zero position" class="DigNum (strict)"() -> ("Value"=w366:dbl)  [unwired: 2 in, 2 out]
                    n249 = property on="Go0" class="Bool (strict)"("Value"=FALSE ("Go2")) -> ()  [unwired: 2 in, 2 out]
                    n250 = property on="Units" class="CmbBox"() -> ("Value"=w367:string)  [unwired: 2 in, 2 out]
                    n251 = case shown="\"lam\"" w367 {
                      tunnel: [w372 w374 w377 w380] -> w368
                      tunnel: w366 -> [w372 w373 w376 w379]
                      frame "mm", Default {
                      }
                      frame "um" {
                        n252 = Multiply(x=w373, y=0.001) -> (x*y=w374:dbl)
                      }
                      frame "nm" {
                        n253 = Multiply(x=w376, y=1e-06) -> (x*y=w377:dbl)
                      }
                      frame "lam" {
                        n254 = Divide(x=w379, y=1000000.0) -> (x/y=w382:dbl)
                        n255 = property on="lambda" class="DigNum (strict)"() -> ("Value"=w381:dbl)  [unwired: 2 in, 2 out]
                        n256 = Multiply(x=w382, y=w381) -> (x*y=w380:dbl)
                      }
                    }
                    n257 = call <userlib>:"CONEX-CC Absolute Move v2.vi"("Target position"=w368, "Connection Cluster in"=w369) -> ("Connection Cluster out"=w370:T6)  [unwired: 5 in, 2 out]
                  }
                  event "Tare": Value Change {
                    n258 = event-data() -> ()  [unwired: 2 out]
                    n259 = property on="Tare" class="Bool (strict)"("Value"=FALSE ("Tare")) -> ()  [unwired: 2 in, 2 out]
                    n260 = property on="Current position" class="DigNum (strict)"() -> ("Value"=w384:dbl)  [unwired: 2 in, 2 out]
                    n261 = property on="Zero position" class="DigNum (strict)"("Value"=w384) -> ()  [unwired: 2 in, 2 out]
                  }
                  event "Cycle": Value Change {
                    (unwired) 0 ("Numérique")
                    n262 = event-data() -> ()  [unwired: 2 out]
                    n263 = property on="Cycle" class="Bool (strict)"("Value"=TRUE ("Cycle")) -> ()  [unwired: 2 in, 2 out]
                  }
                  event "Units": Value Change {
                    n264 = event-data() -> ("NewVal"=w395:string, "OldVal"=w394:string)  [unwired: 1 out]
                    n265 = property on="(1) Go to:" class="DigNum (strict)"("Caption.Text"=w395) -> ()  [unwired: 2 in, 2 out]
                    n266 = property on="(2) Go to:" class="DigNum (strict)"("Caption.Text"=w395) -> ()  [unwired: 2 in, 2 out]
                    n267 = property on="Step:" class="DigNum (strict)"("Caption.Text"=w395) -> ()  [unwired: 2 in, 2 out]
                    n268 = property on="Current position" class="DigNum (strict)"("Caption.Text"=w395) -> ()  [unwired: 2 in, 2 out]
                    n269 = property on="Relative position" class="DigNum (strict)"("Caption.Text"=w395) -> ()  [unwired: 2 in, 2 out]
                    n270 = property on="Zero position" class="DigNum (strict)"("Caption.Text"=w395) -> ()  [unwired: 2 in, 2 out]
                    n271 = case shown="\"mm\", Default" w394 {
                      tunnel: [1000000.0 ("y") 1000.0 ("y") 1.0 ("y") w400] -> w393
                      frame "mm", Default {
                      }
                      frame "um" {
                      }
                      frame "nm" {
                      }
                      frame "lam" {
                        n272 = property on="lambda" class="DigNum (strict)"() -> ("Value"=w400:dbl)  [unwired: 2 in, 2 out]
                      }
                    }
                    n273 = case shown="\"lam\"" w395 {
                      tunnel: [1000000.0 ("y") 1000.0 ("y") 1.0 ("y") w404] -> w392
                      frame "mm", Default {
                      }
                      frame "um" {
                      }
                      frame "nm" {
                      }
                      frame "lam" {
                        n274 = property on="lambda" class="DigNum (strict)"() -> ("Value"=w404:dbl)  [unwired: 2 in, 2 out]
                      }
                    }
                    n275 = property on="Zero position" class="DigNum (strict)"() -> ("Value"=w390:dbl)  [unwired: 2 in, 2 out]
                    n276 = Divide(x=w393, y=w392) -> (x/y=w391:dbl)
                    n277 = Multiply(x=w390, y=w391) -> (x*y=w389:dbl)
                    n278 = property on="Zero position" class="DigNum (strict)"("Value"=w389) -> ()  [unwired: 2 in, 2 out]
                  }
                }
              }
              n279 = node-c288(w80) -> ()  [unwired: 1 out]
              n280 = node-c288(w82) -> ()  [unwired: 1 out]
              n281 = Unbundle By Name(w77) -> ("VISA resource name"=w76:refnum<visa-resource-name>, "error"=w75:errorcluster)
            }
            frame #3 {
            }
          }
        }
      }
      n282 = call <userlib>:"_Close Communications.vi"("Instrument Channel"=w21) -> ()  [unwired: 14 in, 1 out]
      n283 = call <vilib>:"Simple Error Handler.vi"("error in (no error)"=w25) -> ()  [unwired: 1 in, 8 out]
      n284 = call <vilib>:"Simple Error Handler.vi"("error in (no error)"=w14) -> ()  [unwired: 1 in, 8 out]
      n285 = call <vilib>:"Simple Error Handler.vi"("error in (no error)"=w15) -> ()  [unwired: 1 in, 8 out]
    }
  }
